vi "Read Feed forward ref.vi"(8 "error in (no error)":errorcluster, 11 "FpgaRef5782 in":refnum<class "FpgaRef5782.lvclass">) -> (0 "error out":errorcluster, 2 "Feed forward ref":T1, 3 "FpgaRef5782 out":refnum<class "FpgaRef5782.lvclass">)   [LabVIEW 2018, in "FpgaRef5782.lvclass"]
uses:
  FpgaRef5782.lvclass
  Scope5782/Config/FPGAref_5782_FeedForward.ctl
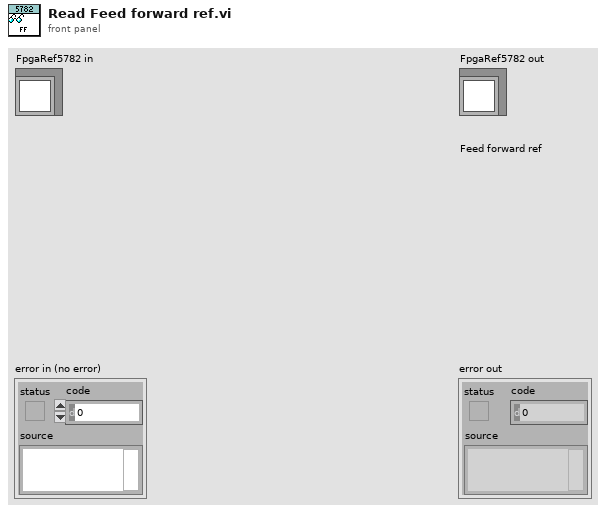
[diagram p1: front panel]
types:
  T1 = typedef "FPGAref_5782_FeedForward.ctl" = refnum<k20>
  T2 = typedef "5782 FPGA ref.ctl" = refnum<k20>
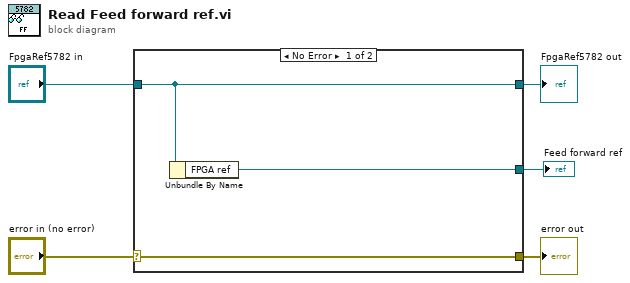
[diagram p0: block diagram]
diagram:
  n1 = case shown="No Error" "error in (no error)" {
    selector: "error in (no error)" -> [w8 w9]
    tunnel: [w8 w9] -> w4
    tunnel: [w7 w10] -> w2
    tunnel: "FpgaRef5782 in" -> [w7 w10]
    tunnel: [w6 _] -> w1
    frame No Error {
      n2 = Unbundle By Name(w7) -> ("FPGA ref"=w6:T2)
    }
    frame Error {
    }
  }
  "error out" <- w4
  "FpgaRef5782 out" <- w2
  "Feed forward ref" <- w1
